vi "MGCC_StaEst_submain.vi"(0 "V_node":cdb[][](array[numeric]), 1 "I_node":cdb[][](array[numeric]), 2 "vbase":dbl=6928.4, 3 "sspn":dbl[][](array[numeric]), 4 "ssqn":dbl[][](array[numeric]), 5 "P_node":cdb[][](array[numeric]), 6 "ssvn":dbl[][](array[numeric]), 7 "Topology":dbl[][](array[numeric]), 9 "NumN":dbl, 11 "NumL":dbl, 12 "Ybus":cdb[][](array[numeric]), 15 "interrupt":dbl=1.0) -> (8 "VN":dbl[][](array[numeric]), 10 "error out":errorcluster, 14 "AN":dbl[][](array[numeric]))   [LabVIEW 2016]
doc: "-----------------------------------------------------------------------------------------------------------------------\nCopyright <2019> <The University of Tennessee at Knoxville and the University of Tennessee Research Foundation>\nThis software is released under BSD-3 \nhttps://opensource.org/licenses/BSD-3-Clause \nAdditional license options available at https://utrf.tennessee.edu/industry/sample-agreements/\n-----------------------------------------------------------------------------------------------------------------------"
uses:
  <vilib>/Utility/error.llb/Error Cluster From Error Code.vi
  Model Management/Global_MdlMgmt.vi
  <vilib>/imath/engines/lvmath2/RunTimeSupport/NIMS_Error if Not Equal.vi
  <instcachedir>/0/NIMS_Error if Not Equal_43252A79AD05436189442EC0C5E5AB8A.lvgen/NIMS_Error if Not Equal_43252A79AD05436189442EC0C5E5AB8A_000.vi
  <vilib>/imath/engines/lvmath2/RunTimeEngine/IndexRead/NIMS M(S,S).vi
  <instcachedir>/0/NIMS M(S,S)_AC51E74150A542F7991B9634C66F3096.lvgen/NIMS M(S,S)_AC51E74150A542F7991B9634C66F3096_001.vi
  <vilib>/imath/engines/lvmath2/RunTimeEngine/BuiltInFunctions/abs/NIMS_abs(signed).vi
  <instcachedir>/0/NIMS_abs(signed)_C4FCB8E6058B49B797C7C8D53CA5F6EC.lvgen/NIMS_abs(signed)_C4FCB8E6058B49B797C7C8D53CA5F6EC_002.vi
  <vilib>/imath/engines/lvmath2/RunTimeEngine/RunTimeType/NIMS_RunTimeType_From StrictType (excl LVString).vi
  <instcachedir>/0/NIMS_RunTimeType_From StrictType (excl LVString)_BBF44FB49F834B71AF7A14CCEDF8BECD.lvgen/NIMS_RunTimeType_From StrictType (excl LVString)_BBF44FB49F834B71AF7A14CCEDF8BECD_031.vi
  <vilib>/imath/engines/lvmath2/RunTimeEngine/Struct/NIMS_StructSetField.vi
  <vilib>/imath/engines/lvmath2/RunTimeEngine/ErrorHandling/NIMS_Create Error From Enums.vi
  <instcachedir>/0/NIMS_RunTimeType_From StrictType (excl LVString)_BBF44FB49F834B71AF7A14CCEDF8BECD.lvgen/NIMS_RunTimeType_From StrictType (excl LVString)_BBF44FB49F834B71AF7A14CCEDF8BECD_032.vi
  <vilib>/imath/engines/lvmath2/RunTimeEngine/Struct/NIMS_StructGetField.vi
  <vilib>/imath/engines/lvmath2/RunTimeEngine/RunTimeType/NIMS_RunTimeType_To Numeric.vi
  <instcachedir>/0/NIMS_RunTimeType_To Numeric_19D51BCABB82435A94073491761E42EE.lvgen/NIMS_RunTimeType_To Numeric_19D51BCABB82435A94073491761E42EE_010.vi
  <instcachedir>/0/NIMS_RunTimeType_To Numeric_19D51BCABB82435A94073491761E42EE.lvgen/NIMS_RunTimeType_To Numeric_19D51BCABB82435A94073491761E42EE_009.vi
  <instcachedir>/0/NIMS_RunTimeType_From StrictType (excl LVString)_BBF44FB49F834B71AF7A14CCEDF8BECD.lvgen/NIMS_RunTimeType_From StrictType (excl LVString)_BBF44FB49F834B71AF7A14CCEDF8BECD_000.vi
  <instcachedir>/0/NIMS_RunTimeType_To Numeric_19D51BCABB82435A94073491761E42EE.lvgen/NIMS_RunTimeType_To Numeric_19D51BCABB82435A94073491761E42EE_000.vi
  <vilib>/imath/engines/lvmath2/RunTimeEngine/IndexRead/NIMS M($,R2).vi
  <instcachedir>/0/NIMS M($,R2)_D9380E19261A4ADFB2D364AF6959C6EF.lvgen/NIMS M($,R2)_D9380E19261A4ADFB2D364AF6959C6EF_000.vi
  <vilib>/imathl/engines/lvmath/Functions/Error Handling/Create Error.vi
  <instcachedir>/0/NIMS_RunTimeType_From StrictType (excl LVString)_BBF44FB49F834B71AF7A14CCEDF8BECD.lvgen/NIMS_RunTimeType_From StrictType (excl LVString)_BBF44FB49F834B71AF7A14CCEDF8BECD_009.vi
  <vilib>/imath/engines/lvmath2/RunTimeEngine/BuiltInFunctions/imag/NIMS_imag(Complex).vi
  <instcachedir>/0/NIMS_imag(Complex)_3180D40D00C843A49C2B33397F857BF3.lvgen/NIMS_imag(Complex)_3180D40D00C843A49C2B33397F857BF3_001.vi
  <instcachedir>/0/NIMS_abs(signed)_C4FCB8E6058B49B797C7C8D53CA5F6EC.lvgen/NIMS_abs(signed)_C4FCB8E6058B49B797C7C8D53CA5F6EC_003.vi
  <vilib>/imath/engines/lvmath2/RunTimeEngine/BuiltInFunctions/angle/NIMS_angle.vi
  <instcachedir>/0/NIMS_angle_6DDAE2BD99E0421EB990B6436E94D88F.lvgen/NIMS_angle_6DDAE2BD99E0421EB990B6436E94D88F_001.vi
  <instcachedir>/0/NIMS_RunTimeType_To Numeric_19D51BCABB82435A94073491761E42EE.lvgen/NIMS_RunTimeType_To Numeric_19D51BCABB82435A94073491761E42EE_003.vi
  <instcachedir>/0/NIMS_abs(signed)_C4FCB8E6058B49B797C7C8D53CA5F6EC.lvgen/NIMS_abs(signed)_C4FCB8E6058B49B797C7C8D53CA5F6EC_005.vi
  <vilib>/imath/engines/lvmath2/RunTimeEngine/VariableToken/Support/NIMS_Matrix Boolean Index to I32 Index.vi
  <vilib>/imath/engines/lvmath2/RunTimeEngine/IndexReplace/NIMS M(V)=S.vi
  <instcachedir>/0/NIMS M(V)=S_F2304187E1344F60ABCBE5C5CC0920F9.lvgen/NIMS M(V)=S_F2304187E1344F60ABCBE5C5CC0920F9_000.vi
  <instcachedir>/0/NIMS M($,R2)_D9380E19261A4ADFB2D364AF6959C6EF.lvgen/NIMS M($,R2)_D9380E19261A4ADFB2D364AF6959C6EF_001.vi
  <instcachedir>/0/NIMS_RunTimeType_From StrictType (excl LVString)_BBF44FB49F834B71AF7A14CCEDF8BECD.lvgen/NIMS_RunTimeType_From StrictType (excl LVString)_BBF44FB49F834B71AF7A14CCEDF8BECD_024.vi
  LabVIEW Data/MathScriptVIs/MCStatic_36913153632_be44ae6048cc796b65fe61fbcc6124bb.vi
  <instcachedir>/0/MCStatic_36913153632_be44ae6048cc796b65fe61fbcc6124bb_299CCFB54962426892AA262595275464.lvgen/MCStatic_36913153632_be44ae6048cc796b65fe61fbcc6124bb_299CCFB54962426892AA262595275464_000.vi
  <instcachedir>/0/NIMS_RunTimeType_To Numeric_19D51BCABB82435A94073491761E42EE.lvgen/NIMS_RunTimeType_To Numeric_19D51BCABB82435A94073491761E42EE_008.vi
  <vilib>/imath/engines/lvmath2/RunTimeEngine/BuiltInFunctions/size/NIMS_I32=size(GRow,I32).vi
  <instcachedir>/0/NIMS_I32=size(GRow,I32)_ECB8D6BA8B644FAD9EC9BDD2BFE864D8.lvgen/NIMS_I32=size(GRow,I32)_ECB8D6BA8B644FAD9EC9BDD2BFE864D8_000.vi
  <vilib>/imath/engines/lvmath2/RunTimeEngine/RangeToken/NIMS_Range_R2 - Integer.vi
  <instcachedir>/0/NIMS_Range_R2 - Integer_89B873E74E6E489885E44F751DD9C6BF.lvgen/NIMS_Range_R2 - Integer_89B873E74E6E489885E44F751DD9C6BF_000.vi
  <vilib>/imath/engines/lvmath2/RunTimeEngine/CommandStatement/MC_CommandStatement_break.vi
  <vilib>/imath/engines/lvmath2/RunTimeEngine/IndexRead/NIMS M(S).vi
  <instcachedir>/0/NIMS M(S)_B826C018497E4940AE96BD27B540B6FB.lvgen/NIMS M(S)_B826C018497E4940AE96BD27B540B6FB_000.vi
  <vilib>/imath/engines/lvmath2/RunTimeEngine/MatrixToken/NIMS_MatrixToken_M_RV.vi
  <instcachedir>/0/NIMS_MatrixToken_M_RV_EE14907D4B194E829889005D2F556E9C.lvgen/NIMS_MatrixToken_M_RV_EE14907D4B194E829889005D2F556E9C_001.vi
  LabVIEW Data/MathScriptVIs/MCStatic_36913153632_768d10d24ec5cae2ef0a1ce42dd6f61b.vi
  <instcachedir>/0/MCStatic_36913153632_768d10d24ec5cae2ef0a1ce42dd6f61b_42FB18720A4D4D57895E758F2AD9E816.lvgen/MCStatic_36913153632_768d10d24ec5cae2ef0a1ce42dd6f61b_42FB18720A4D4D57895E758F2AD9E816_000.vi
  <vilib>/imath/engines/lvmath2/RunTimeEngine/RangeToken/NIMS_Range.vi
  <instcachedir>/0/NIMS_Range_A7C094595B484CA7AF10685B02D808ED.lvgen/NIMS_Range_A7C094595B484CA7AF10685B02D808ED_000.vi
  <instcachedir>/0/NIMS_RunTimeType_From StrictType (excl LVString)_BBF44FB49F834B71AF7A14CCEDF8BECD.lvgen/NIMS_RunTimeType_From StrictType (excl LVString)_BBF44FB49F834B71AF7A14CCEDF8BECD_010.vi
  <instcachedir>/0/NIMS_RunTimeType_To Numeric_19D51BCABB82435A94073491761E42EE.lvgen/NIMS_RunTimeType_To Numeric_19D51BCABB82435A94073491761E42EE_004.vi
  <vilib>/imath/engines/lvmath2/RunTimeEngine/BuiltInFunctions/length/NIMS_length(GV).vi
  <instcachedir>/0/NIMS_length(GV)_08A3D13377FD4E4B96F5795FBF3698FA.lvgen/NIMS_length(GV)_08A3D13377FD4E4B96F5795FBF3698FA_000.vi
  <vilib>/imath/engines/lvmath2/RunTimeEngine/BuiltInFunctions/size/NIMS_I32Row=size(GCol).vi
  <instcachedir>/0/NIMS_I32Row=size(GCol)_6F63159FA7824881BFA06400543D6D03.lvgen/NIMS_I32Row=size(GCol)_6F63159FA7824881BFA06400543D6D03_000.vi
  <vilib>/imath/engines/lvmath2/RunTimeEngine/RangeToken/NIMS_Range_R3 - Integer.vi
  <instcachedir>/0/NIMS_Range_R3 - Integer_A435E2FF893B4C718FD5055FE39FE2F6.lvgen/NIMS_Range_R3 - Integer_A435E2FF893B4C718FD5055FE39FE2F6_000.vi
  <vilib>/imath/engines/lvmath2/RunTimeEngine/IndexRead/NIMS V(S).vi
  <instcachedir>/0/NIMS V(S)_0488751826AF41519A22953C041130DC.lvgen/NIMS V(S)_0488751826AF41519A22953C041130DC_000.vi
  <vilib>/imath/engines/lvmath2/RunTimeEngine/IndexReplace/NIMS V(S)=S.vi
  <instcachedir>/0/NIMS V(S)=S_57E16554CB8B4B90AAB163894F717546.lvgen/NIMS V(S)=S_57E16554CB8B4B90AAB163894F717546_000.vi
  LabVIEW Data/MathScriptVIs/MCStatic_36913153632_1e6ad96140824169305d556de171d12e.vi
  <instcachedir>/0/MCStatic_36913153632_1e6ad96140824169305d556de171d12e_64F75552A8F844369C23CF330D52EDD5.lvgen/MCStatic_36913153632_1e6ad96140824169305d556de171d12e_64F75552A8F844369C23CF330D52EDD5_000.vi
  <instcachedir>/0/NIMS_Error if Not Equal_43252A79AD05436189442EC0C5E5AB8A.lvgen/NIMS_Error if Not Equal_43252A79AD05436189442EC0C5E5AB8A_001.vi
  <vilib>/imath/engines/lvmath2/RunTimeEngine/IndexRead/NIMS M(V,R2).vi
  <instcachedir>/0/NIMS M(V,R2)_C347351B41664C5DBDDF0EFBABEC5506.lvgen/NIMS M(V,R2)_C347351B41664C5DBDDF0EFBABEC5506_000.vi
  <vilib>/imath/engines/lvmath2/RunTimeEngine/ArithmeticOperatorToken/NIMS_ArithmeticOperator_times.vi
  <instcachedir>/0/NIMS_ArithmeticOperator_times_953B34F74CAC448FB707D816A29CC5F0.lvgen/NIMS_ArithmeticOperator_times_953B34F74CAC448FB707D816A29CC5F0_007.vi
  <vilib>/imath/engines/lvmath2/RunTimeEngine/BuiltInFunctions/reshapemx/NIMS_[GV]_reshapemx.vi
  <instcachedir>/0/NIMS_[GV]_reshapemx_314E456D64644EB191D4916921E89AA6.lvgen/NIMS_[GV]_reshapemx_314E456D64644EB191D4916921E89AA6_000.vi
  <vilib>/imath/engines/lvmath2/RunTimeEngine/IndexRead/NIMS M(V,S).vi
  <instcachedir>/0/NIMS M(V,S)_4A7282EC9BD94252BB5D44AC841A97D6.lvgen/NIMS M(V,S)_4A7282EC9BD94252BB5D44AC841A97D6_000.vi
  <vilib>/imath/engines/lvmath2/RunTimeEngine/IndexRead/NIMS M($,S).vi
  <instcachedir>/0/NIMS M($,S)_3E5749BBB62E49528D4765A77F1F6D98.lvgen/NIMS M($,S)_3E5749BBB62E49528D4765A77F1F6D98_000.vi
  <vilib>/imath/engines/lvmath2/RunTimeEngine/BuiltInFunctions/size/NIMS_I32Row=size(GRow).vi
  <instcachedir>/0/NIMS_I32Row=size(GRow)_E5C05C6B13124B29B774CC4F993D3C59.lvgen/NIMS_I32Row=size(GRow)_E5C05C6B13124B29B774CC4F993D3C59_000.vi
  <vilib>/imath/engines/lvmath2/RunTimeEngine/BuiltInFunctions/ones/NIMS_M=ones(I32V).vi
  <vilib>/imath/engines/lvmath2/RunTimeEngine/RowToken/NIMS_RowToken_M_M.vi
  <instcachedir>/0/NIMS_RowToken_M_M_968CDE3545E74ACDAEA4B48DE01EEECA.lvgen/NIMS_RowToken_M_M_968CDE3545E74ACDAEA4B48DE01EEECA_004.vi
  <vilib>/imath/engines/lvmath2/RunTimeEngine/BuiltInFunctions/diag/NIMS_diag.vi
  <instcachedir>/0/NIMS_diag_BAFF033CE85645D0951408836EA255EA.lvgen/NIMS_diag_BAFF033CE85645D0951408836EA255EA_003.vi
  <vilib>/imath/engines/lvmath2/RunTimeEngine/RowToken/NIMS_RowToken_CV_CV.vi
  <instcachedir>/0/NIMS_RowToken_CV_CV_5546A0B1CA2C4E49826F811B9C073FB0.lvgen/NIMS_RowToken_CV_CV_5546A0B1CA2C4E49826F811B9C073FB0_000.vi
  <vilib>/imath/engines/lvmath2/RunTimeEngine/BuiltInFunctions/zeros/NIMS_M=zeros(I32,I32).vi
  <vilib>/imath/engines/lvmath2/RunTimeEngine/RangeToken/NIMS_Range_R2 - Float.vi
  <instcachedir>/0/NIMS_Range_R2 - Float_590A1087448447AEB7F770FC082D3801.lvgen/NIMS_Range_R2 - Float_590A1087448447AEB7F770FC082D3801_000.vi
  <vilib>/imath/engines/lvmath2/RunTimeEngine/IndexReplace/NIMS M(S,S)=S.vi
  <instcachedir>/0/NIMS M(S,S)=S_98E40400474E4398B113AE20298B4F82.lvgen/NIMS M(S,S)=S_98E40400474E4398B113AE20298B4F82_000.vi
  LabVIEW Data/MathScriptVIs/MCStatic_36913153632_6298f8f6c83752723d2226ea016fc197.vi
  <instcachedir>/0/MCStatic_36913153632_6298f8f6c83752723d2226ea016fc197_3642FD24B40E4351BB90101570A96C12.lvgen/MCStatic_36913153632_6298f8f6c83752723d2226ea016fc197_3642FD24B40E4351BB90101570A96C12_000.vi
  LabVIEW Data/MathScriptVIs/MCStatic_36913153632_74b80caf5031e046e71450c869b25ac4.vi
  <instcachedir>/0/MCStatic_36913153632_74b80caf5031e046e71450c869b25ac4_EBBE0D165A1844C19D15217B3971A6C8.lvgen/MCStatic_36913153632_74b80caf5031e046e71450c869b25ac4_EBBE0D165A1844C19D15217B3971A6C8_000.vi
  <vilib>/imath/engines/lvmath2/RunTimeEngine/MatrixToken/NIMS_MatrixToken_M_M.vi
  <instcachedir>/0/NIMS_MatrixToken_M_M_DF273B0CC20F424BBF1EDA9F4E71C841.lvgen/NIMS_MatrixToken_M_M_DF273B0CC20F424BBF1EDA9F4E71C841_004.vi
  <vilib>/imath/engines/lvmath2/RunTimeEngine/IndexReplace/NIMS M($,V)=S.vi
  <instcachedir>/0/NIMS M($,V)=S_8FF4B0FF94A24B3598424F2A899DBD06.lvgen/NIMS M($,V)=S_8FF4B0FF94A24B3598424F2A899DBD06_000.vi
  LabVIEW Data/MathScriptVIs/MCStatic_36913153632_b1439afdde66222fcd04c55d7a6778ce.vi
  <instcachedir>/0/MCStatic_36913153632_b1439afdde66222fcd04c55d7a6778ce_EEE05774F8294989AC0FB7279B922BFB.lvgen/MCStatic_36913153632_b1439afdde66222fcd04c55d7a6778ce_EEE05774F8294989AC0FB7279B922BFB_000.vi
  LabVIEW Data/MathScriptVIs/MCStatic_36913153632_4de716850640586bd02f98b625ef993e.vi
  <instcachedir>/0/MCStatic_36913153632_4de716850640586bd02f98b625ef993e_4E7D4A7640E146149C2F9063A07B5FB8.lvgen/MCStatic_36913153632_4de716850640586bd02f98b625ef993e_4E7D4A7640E146149C2F9063A07B5FB8_000.vi
  <vilib>/imath/engines/lvmath2/RunTimeEngine/ArithmeticOperatorToken/NIMS_ArithmeticOperator_minus.vi
  <instcachedir>/0/NIMS_ArithmeticOperator_minus_E3B65B1D26A44BB184AFDC5B3F458E3D.lvgen/NIMS_ArithmeticOperator_minus_E3B65B1D26A44BB184AFDC5B3F458E3D_003.vi
  <vilib>/imath/engines/lvmath2/RunTimeEngine/ArithmeticOperatorToken/NIMS_ArithmeticOperator_rightdivmx.vi
  <instcachedir>/0/NIMS_ArithmeticOperator_rightdivmx_0DBBD6F2821B4AB59571CD9AB2DE9D62.lvgen/NIMS_ArithmeticOperator_rightdivmx_0DBBD6F2821B4AB59571CD9AB2DE9D62_000.vi
  <vilib>/imath/engines/lvmath2/RunTimeEngine/ArithmeticOperatorToken/NIMS_ArithmeticOperator_multmx(M,CV).vi
  <instcachedir>/0/NIMS_ArithmeticOperator_multmx(M,CV)_EE734FC8520844C9A7CC1A67008668A3.lvgen/NIMS_ArithmeticOperator_multmx(M,CV)_EE734FC8520844C9A7CC1A67008668A3_000.vi
  <vilib>/imath/engines/lvmath2/RunTimeEngine/ArithmeticOperatorToken/NIMS_ArithmeticOperator_multmx.vi
  <instcachedir>/0/NIMS_ArithmeticOperator_multmx_4A56FE5C615140CE835D4DB5891BF065.lvgen/NIMS_ArithmeticOperator_multmx_4A56FE5C615140CE835D4DB5891BF065_004.vi
  <vilib>/imath/engines/lvmath2/RunTimeEngine/BuiltInFunctions/pinv/NIMS_pinv.vi
  <instcachedir>/0/NIMS_pinv_206F0700CF75499C820074BA4F1FFC36.lvgen/NIMS_pinv_206F0700CF75499C820074BA4F1FFC36_000.vi
  <vilib>/imath/engines/lvmath2/RunTimeEngine/ErrorHandling/NIMS_Error From Error Code.vi
  LabVIEW Data/MathScriptVIs/MCStatic_36913153632_4a49c84bbcd428c212b20195cbe8b035.vi
  <instcachedir>/0/MCStatic_36913153632_4a49c84bbcd428c212b20195cbe8b035_991BF795119A46088146E750DEF0BE67.lvgen/MCStatic_36913153632_4a49c84bbcd428c212b20195cbe8b035_991BF795119A46088146E750DEF0BE67_000.vi
  LabVIEW Data/MathScriptVIs/MCStatic_36913153632_a7ddd08330f9b3077b19931b3d4ed570.vi
  <instcachedir>/0/MCStatic_36913153632_a7ddd08330f9b3077b19931b3d4ed570_A5488D48717747F080A6F4A94BE5B924.lvgen/MCStatic_36913153632_a7ddd08330f9b3077b19931b3d4ed570_A5488D48717747F080A6F4A94BE5B924_000.vi
  <instcachedir>/0/NIMS_ArithmeticOperator_minus_E3B65B1D26A44BB184AFDC5B3F458E3D.lvgen/NIMS_ArithmeticOperator_minus_E3B65B1D26A44BB184AFDC5B3F458E3D_002.vi
  <vilib>/imath/engines/lvmath2/RunTimeEngine/BuiltInFunctions/max/1 input/NIMS_max(RM).vi
  <instcachedir>/0/NIMS_max(RM)_358AE92FF7FA4D91BF0D9DEC69043403.lvgen/NIMS_max(RM)_358AE92FF7FA4D91BF0D9DEC69043403_000.vi
  <vilib>/imath/engines/lvmath2/RunTimeEngine/ArithmeticOperatorToken/NIMS_ArithmeticOperator_plus.vi
  <instcachedir>/0/NIMS_ArithmeticOperator_plus_0120E0498A0F4B4B9BDCAC2554767A4E.lvgen/NIMS_ArithmeticOperator_plus_0120E0498A0F4B4B9BDCAC2554767A4E_003.vi
  <vilib>/imath/engines/lvmath2/RunTimeEngine/VariableToken/NIMS_VariableToken_CondDefined.vi
  <instcachedir>/0/NIMS_VariableToken_CondDefined_06E9DA95BD4D46A6BA55EC651A891960.lvgen/NIMS_VariableToken_CondDefined_06E9DA95BD4D46A6BA55EC651A891960_001.vi
  <vilib>/imath/engines/lvmath2/RunTimeEngine/IndexRead/NIMS M(V).vi
  <instcachedir>/0/NIMS M(V)_948FAC22C1C943948B75DA6190348614.lvgen/NIMS M(V)_948FAC22C1C943948B75DA6190348614_005.vi
  <vilib>/imath/engines/lvmath2/RunTimeEngine/BuiltInFunctions/reshapemx/NIMS_[GM]_reshapemx.vi
  <instcachedir>/0/NIMS_[GM]_reshapemx_500BD31B48F5434EA23B2056DCB44201.lvgen/NIMS_[GM]_reshapemx_500BD31B48F5434EA23B2056DCB44201_000.vi
  <instcachedir>/0/NIMS_ArithmeticOperator_plus_0120E0498A0F4B4B9BDCAC2554767A4E.lvgen/NIMS_ArithmeticOperator_plus_0120E0498A0F4B4B9BDCAC2554767A4E_010.vi
  <instcachedir>/0/NIMS_VariableToken_CondDefined_06E9DA95BD4D46A6BA55EC651A891960.lvgen/NIMS_VariableToken_CondDefined_06E9DA95BD4D46A6BA55EC651A891960_004.vi
  <instcachedir>/0/NIMS_VariableToken_CondDefined_06E9DA95BD4D46A6BA55EC651A891960.lvgen/NIMS_VariableToken_CondDefined_06E9DA95BD4D46A6BA55EC651A891960_005.vi
  <vilib>/imath/engines/lvmath/Functions/Error Handling/MergeErrorsWrapper.vi
  <vilib>/imath/engines/lvmath2/RunTimeEngine/NodeEndStatement/NIMS_NodeEndStatement_Output.vi
  <instcachedir>/0/NIMS_NodeEndStatement_Output_53EC0D466D134D7ABD903AC30B43404B.lvgen/NIMS_NodeEndStatement_Output_53EC0D466D134D7ABD903AC30B43404B_002.vi
  <instcachedir>/0/NIMS_NodeEndStatement_Output_53EC0D466D134D7ABD903AC30B43404B.lvgen/NIMS_NodeEndStatement_Output_53EC0D466D134D7ABD903AC30B43404B_005.vi
  <instcachedir>/0/NIMS_NodeEndStatement_Output_53EC0D466D134D7ABD903AC30B43404B.lvgen/NIMS_NodeEndStatement_Output_53EC0D466D134D7ABD903AC30B43404B_025.vi
  <instcachedir>/0/NIMS_NodeEndStatement_Output_53EC0D466D134D7ABD903AC30B43404B.lvgen/NIMS_NodeEndStatement_Output_53EC0D466D134D7ABD903AC30B43404B_011.vi
  <instcachedir>/0/NIMS_NodeEndStatement_Output_53EC0D466D134D7ABD903AC30B43404B.lvgen/NIMS_NodeEndStatement_Output_53EC0D466D134D7ABD903AC30B43404B_024.vi
  <instcachedir>/0/NIMS_NodeEndStatement_Output_53EC0D466D134D7ABD903AC30B43404B.lvgen/NIMS_NodeEndStatement_Output_53EC0D466D134D7ABD903AC30B43404B_003.vi
  <instcachedir>/0/NIMS_NodeEndStatement_Output_53EC0D466D134D7ABD903AC30B43404B.lvgen/NIMS_NodeEndStatement_Output_53EC0D466D134D7ABD903AC30B43404B_001.vi
  <instcachedir>/0/NIMS_NodeEndStatement_Output_53EC0D466D134D7ABD903AC30B43404B.lvgen/NIMS_NodeEndStatement_Output_53EC0D466D134D7ABD903AC30B43404B_023.vi
  <instcachedir>/0/NIMS_NodeEndStatement_Output_53EC0D466D134D7ABD903AC30B43404B.lvgen/NIMS_NodeEndStatement_Output_53EC0D466D134D7ABD903AC30B43404B_022.vi
  <instcachedir>/0/NIMS_NodeEndStatement_Output_53EC0D466D134D7ABD903AC30B43404B.lvgen/NIMS_NodeEndStatement_Output_53EC0D466D134D7ABD903AC30B43404B_021.vi
  <instcachedir>/0/NIMS_NodeEndStatement_Output_53EC0D466D134D7ABD903AC30B43404B.lvgen/NIMS_NodeEndStatement_Output_53EC0D466D134D7ABD903AC30B43404B_020.vi
  <instcachedir>/0/NIMS_NodeEndStatement_Output_53EC0D466D134D7ABD903AC30B43404B.lvgen/NIMS_NodeEndStatement_Output_53EC0D466D134D7ABD903AC30B43404B_019.vi
  <instcachedir>/0/NIMS_NodeEndStatement_Output_53EC0D466D134D7ABD903AC30B43404B.lvgen/NIMS_NodeEndStatement_Output_53EC0D466D134D7ABD903AC30B43404B_018.vi
  <instcachedir>/0/NIMS_NodeEndStatement_Output_53EC0D466D134D7ABD903AC30B43404B.lvgen/NIMS_NodeEndStatement_Output_53EC0D466D134D7ABD903AC30B43404B_017.vi
  <instcachedir>/0/NIMS_NodeEndStatement_Output_53EC0D466D134D7ABD903AC30B43404B.lvgen/NIMS_NodeEndStatement_Output_53EC0D466D134D7ABD903AC30B43404B_004.vi
  <instcachedir>/0/NIMS_NodeEndStatement_Output_53EC0D466D134D7ABD903AC30B43404B.lvgen/NIMS_NodeEndStatement_Output_53EC0D466D134D7ABD903AC30B43404B_027.vi
  <vilib>/imath/engines/lvmath2/RunTimeEngine/ErrorHandling/NIMS_Finalize Error.vi
  <vilib>/imath/engines/lvmath2/RunTimeEngine/RelationalOperatorToken/NIMS_Relational_Operator_Eq.vi
  <instcachedir>/0/NIMS_Relational_Operator_Eq_FD198F059617437A8A02361002FCA645.lvgen/NIMS_Relational_Operator_Eq_FD198F059617437A8A02361002FCA645_003.vi
  <instcachedir>/0/NIMS_NodeEndStatement_Output_53EC0D466D134D7ABD903AC30B43404B.lvgen/NIMS_NodeEndStatement_Output_53EC0D466D134D7ABD903AC30B43404B_015.vi
  <vilib>/ErrorRing/Error Ring.xnode
  cequ.m
  cjoc.m
  idx2pha.m
  pha2idx.m
  pnequ.m
  pnjoc.m
  vnequ.m
  vnjoc.m
  zeroinjec.m
  <instcachedir>/0/MCStatic_36913153632_4de716850640586bd02f98b625ef993e_4E7D4A7640E146149C2F9063A07B5FB8.lvgen/MCStatic_36913153632_4de716850640586bd02f98b625ef993e_4E7D4A7640E146149C2F9063A07B5FB8_001.vi
  <instcachedir>/0/MCStatic_36913153632_6298f8f6c83752723d2226ea016fc197_3642FD24B40E4351BB90101570A96C12.lvgen/MCStatic_36913153632_6298f8f6c83752723d2226ea016fc197_3642FD24B40E4351BB90101570A96C12_001.vi
  <instcachedir>/0/MCStatic_36913153632_74b80caf5031e046e71450c869b25ac4_EBBE0D165A1844C19D15217B3971A6C8.lvgen/MCStatic_36913153632_74b80caf5031e046e71450c869b25ac4_EBBE0D165A1844C19D15217B3971A6C8_001.vi
  <instcachedir>/0/MCStatic_36913153632_a7ddd08330f9b3077b19931b3d4ed570_A5488D48717747F080A6F4A94BE5B924.lvgen/MCStatic_36913153632_a7ddd08330f9b3077b19931b3d4ed570_A5488D48717747F080A6F4A94BE5B924_001.vi
  <instcachedir>/0/MCStatic_36913153632_b1439afdde66222fcd04c55d7a6778ce_EEE05774F8294989AC0FB7279B922BFB.lvgen/MCStatic_36913153632_b1439afdde66222fcd04c55d7a6778ce_EEE05774F8294989AC0FB7279B922BFB_001.vi
panel:
  out "H":dbl[][](array[numeric])
  out "InitialValue":dbl[](array[numeric])
  out "StateVar":dbl[][](array[numeric])
  out "Weight":dbl[][](array[numeric])
  out "Num":T1
  out "B":dbl[][](array[numeric])
  out "MeaPha":T2
  out "Loc":cluster{"Zeroinj":i32[][], "Line":dbl[][]}
  out "pha_rupter":i32[][](array[numeric])
  out "puTrue":T3
  out "Mea":T2
  out "measure":dbl[](array[numeric])
  out "G":dbl[][](array[numeric])
  out "V_node 2":cdb[][](array[numeric])
  out "MeaIdx":cluster{"PN":dbl[], "QN":dbl[], "VN":dbl[]}
  out "idx_rupter":dbl[](array[numeric])
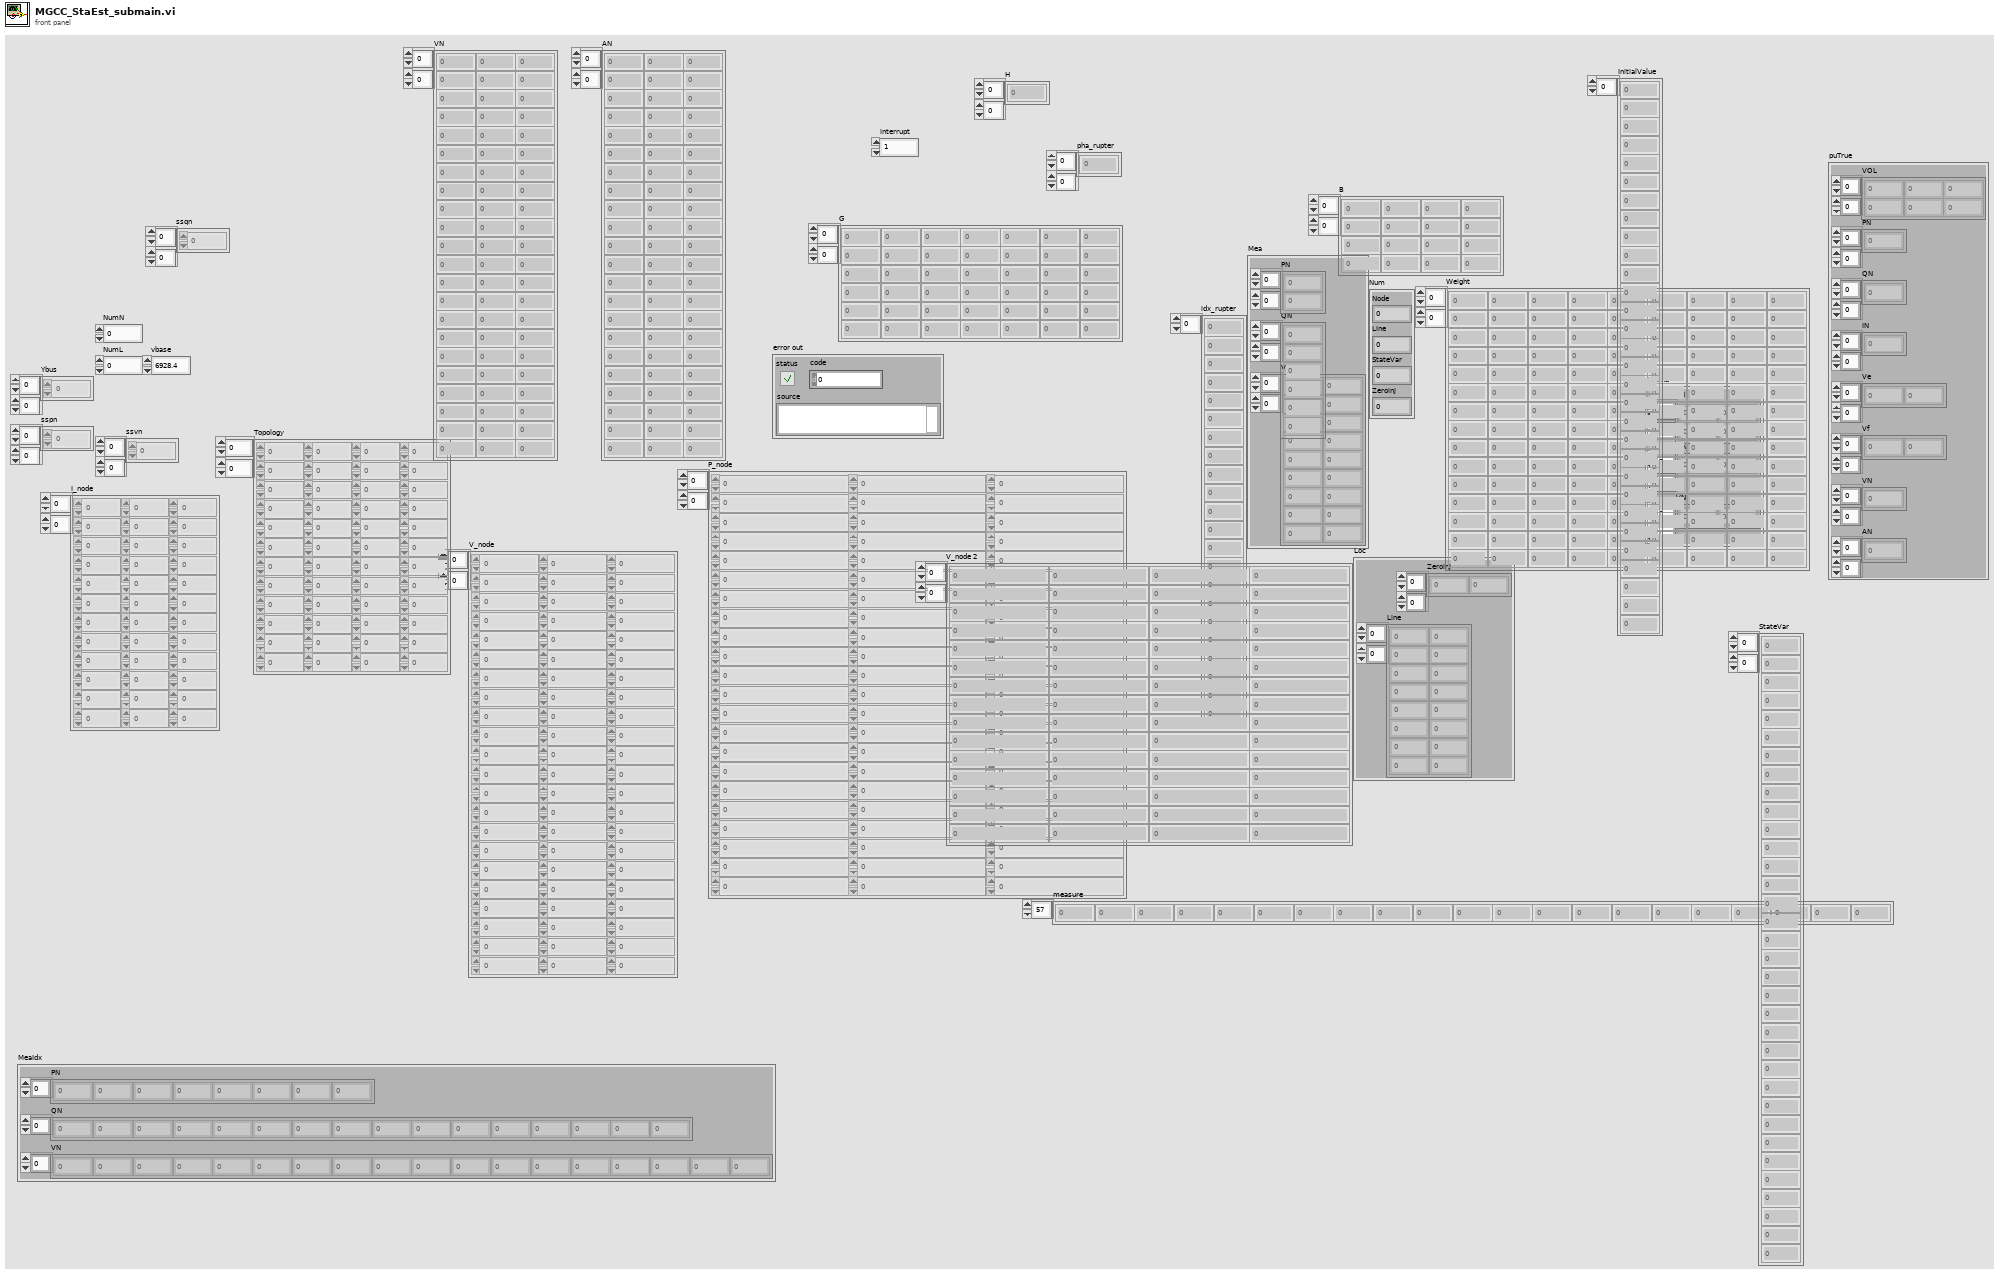
[diagram p1: front panel]
types:
  T1 = cluster{"Node":dbl, "Line":dbl, "StateVar":i32, "Zeroinj":i32}
  T2 = cluster{"PN":dbl[][], "QN":dbl[][], "VN":dbl[][]}
  T3 = cluster{"VOL":cdb[][], "PN":dbl[][], "QN":dbl[][], "IN":dbl[][], "Ve":dbl[][], "Vf":dbl[][], "VN":dbl[][], "AN":dbl[][]}
  T4 = cluster{"Ve":dbl[][], "Vf":dbl[][], "VOL":cdb[][], "AN":dbl[][], "VN":dbl[][]}
  T5 = cluster{"Sbase":dbl, "Vbase":i32, "Ibase":dbl, "Ybase":dbl}
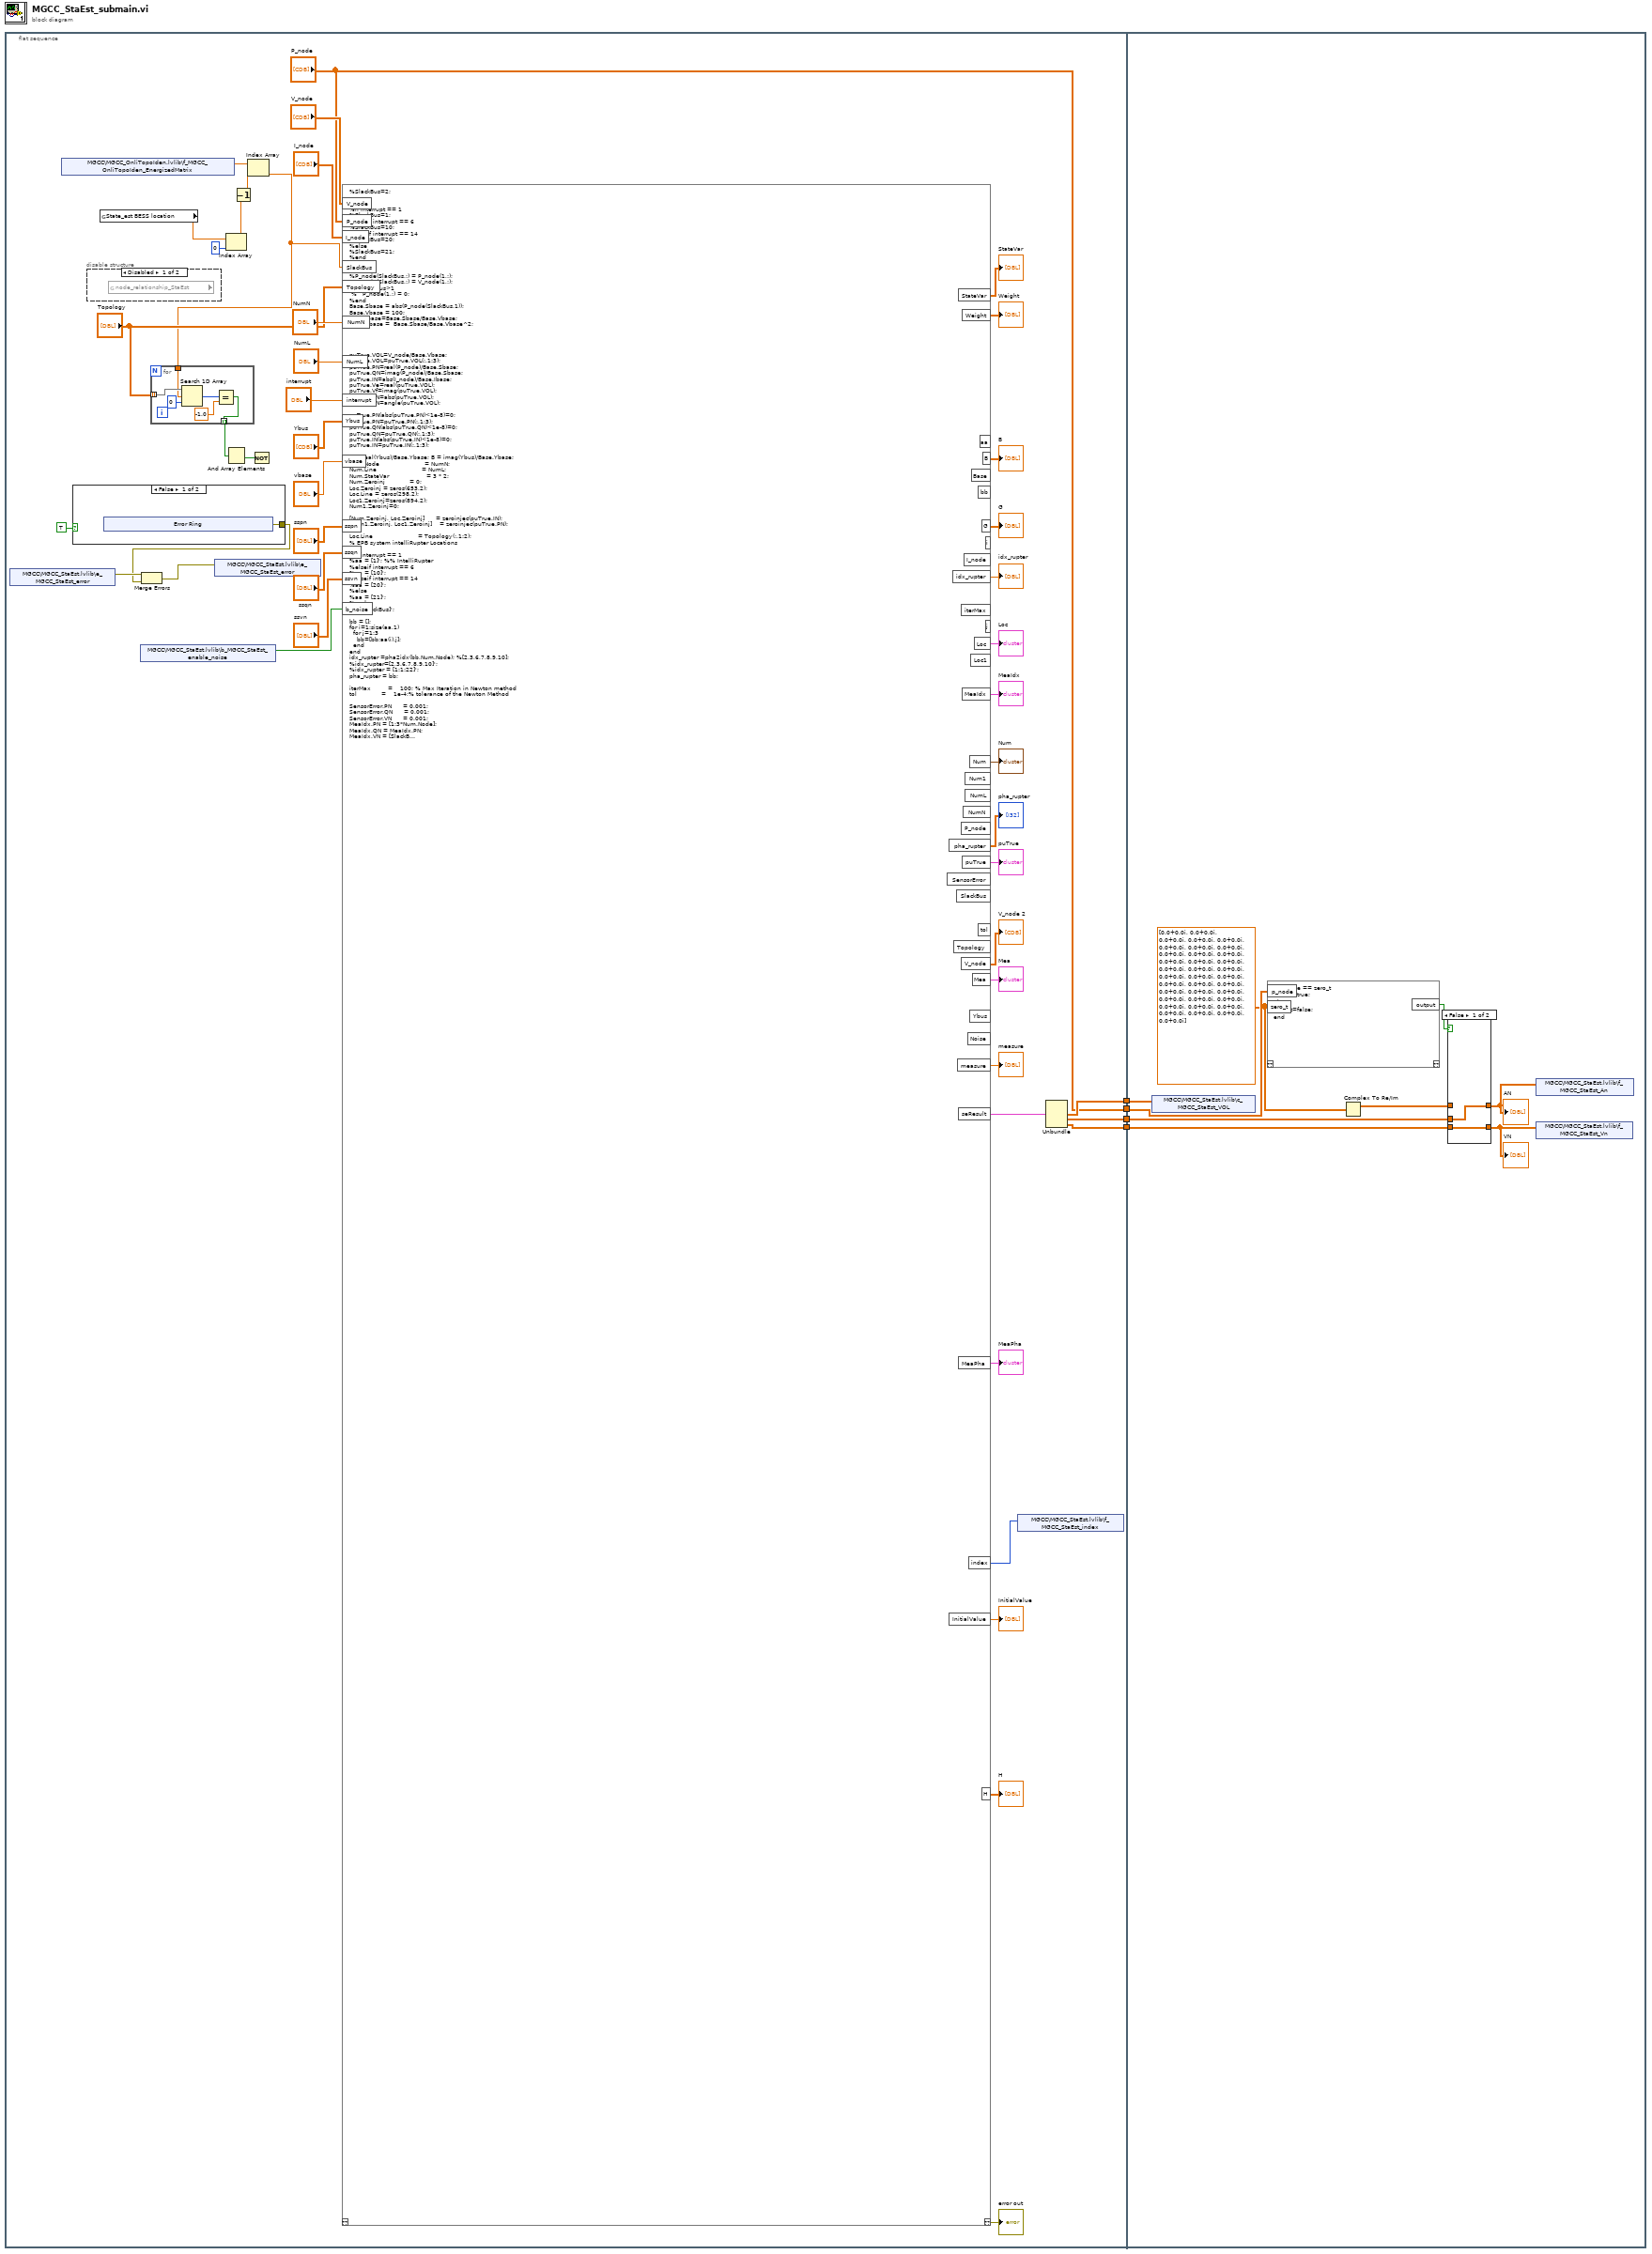
[diagram p0: block diagram]
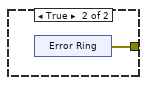
[diagram p2: hidden frame]
diagram:
  n1 = flat-sequence {
    tunnel: [w37] -> w4
    tunnel: ["P_node"] -> w3
    tunnel: [w22] -> w2
    tunnel: [w21] -> w1
    tunnel: w4 -> [w3950]
    tunnel: w3 -> [w3949]
    tunnel: w2 -> [w3946]
    tunnel: w1 -> [w3948]
    frame #0 {
      n2 = shared-variable "MGCC\\MGCC_StaEst.lvlib\\e_MGCC_StaEst_error"() -> (w8:errorcluster)  [unwired: 1 in, 1 out]
      n3 = shared-variable "MGCC\\MGCC_OnliTopoIden.lvlib\\f_MGCC_OnliTopoIden_EnergizedMatrix"() -> (w18:dbl[])  [unwired: 1 in, 1 out]
      n4 = case shown="False" TRUE {
        tunnel: [w52 w58] -> w6
        frame False {
          n5 = xnode "Error Ring"() -> ("error out"=w52:errorcluster)
        }
        frame True {
          n6 = xnode "Error Ring"() -> ("error out"=w58:errorcluster)
        }
      }
      n7 = disable-structure shown="Disabled" {
        frame Disabled {
          n8 = global read "Global_MdlMgmt.vi" "node_relationship_StaEst"() -> ()  [unwired: 1 out]
        }
        frame Enabled {
        }
      }
      n9 = global read "Global_MdlMgmt.vi" "State_est BESS location"() -> (w17:dbl[])
      n10 = shared-variable "MGCC\\MGCC_StaEst.lvlib\\b_MGCC_StaEst_enable_noise"() -> (w38:bool)  [unwired: 1 in, 1 out]
      n11 = Merge Errors(w8, w6) -> (w7:errorcluster)
      n12 = shared-variable "MGCC\\MGCC_StaEst.lvlib\\e_MGCC_StaEst_error"(w7) -> ()  [unwired: 1 in, 1 out]
      n13 = Index Array(array=w17, index=0) -> (element=w15:dbl)
      n14 = Decrement(x=w15) -> (x-1=w14:dbl)
      n15 = Index Array(array=w18, index=w14) -> (element=w11:dbl)
      n16 = for {
        tunnel: "Topology" -> [w65] mode=indexing
        tunnel: w11 -> [w64]
        tunnel: [w60] -> w10 mode=indexing
        n17 = Search 1D Array(1D array=w65, element=w64, start index (0)=0) -> (index of element=w61:i32)
        n18 = Equal?(x=w61, y=-1.0) -> (x = y?=w60:bool)
      }
      n19 = And Array Elements(Boolean array=w10) -> (logical AND=w9:bool)
      n20 = Not(x=w9) -> ()  [unwired: 1 out]
      n21 = mathscript code="%SlackBus=2;\n\n\n%if interrupt == 1\n%SlackBus=1;\n%elseif interrupt == 6\n%SlackBus=10;\n%elseif interrupt == 14\n%SlackBus=20;\n%else\n%SlackBus=21;\n%end\n\n\n%P_node(SlackBus,:) = P_node(1,:);\n%V_node(SlackBus,:) = V_node(1,:);\n%if SlackBus>1\n %   P_node(1,:) = 0;\n%end\nBase.Sbase = abs(P_node(SlackBus,1));\nBase.Vbase = 100;\nBase.Ibase=Base.Sbase/Base.Vbase;\nBase.Ybase =  Base.Sbase/Base.Vbase^2;\n\n\n\n\npuTrue.VOL=V_node/Base.Vbase;\npuTrue.VOL=puTrue.VOL(:,1:3);\npuTrue.PN=real(P_node)/Base.Sbase;\npuTrue.QN=imag(P_node)/Base.Sbase;\npuTrue.IN=abs(I_node)/Base.Ibase;\npuTrue.Ve=real(puTrue.VOL);\npuTrue.Vf=imag(puTrue.VOL); \npuTrue.VN=abs(puTrue.VOL);\npuTrue.AN=angle(puTrue.VOL);\n\npuTrue.PN(abs(puTrue.PN)<1e-8)=0;\npuTrue.PN=puTrue.PN(:,1:3);\npuTrue.QN(abs(puTrue.QN)<1e-8)=0;\npuTrue.QN=puTrue.QN(:,1:3);\npuTrue.IN(abs(puTrue.IN)<1e-8)=0;\npuTrue.IN=puTrue.IN(:,1:3);\n\nG = real(Ybus)/Base.Ybase; B = imag(Ybus)/Base.Ybase;\nNum.Node                        = NumN;\nNum.Line                        = NumL;\nNum.StateVar                    = 3 * 2;  \nNum.Zeroinj             = 0;\nLoc.Zeroinj = zeros(653,2);\nLoc.Line = zeros(298,2);\nLoc1.Zeroinj=zeros(894,2);\nNum1.Zeroinj=0;\n\n[Num.Zeroinj, Loc.Zeroinj]      = zeroinjec(puTrue.IN);\n[Num1.Zeroinj, Loc1.Zeroinj]    = zeroinjec(puTrue.PN);\n\nLoc.Line                        = Topology(:,1:2);\n% EPB system intelliRupter Locations\n\n%if interrupt == 1\n%aa = [1]'; %% IntelliRupter\n%elseif interrupt == 6\n%aa = [10]';\n%elseif interrupt == 14\n%aa = [20]';\n%else\n%aa = [21]';\n%end\naa=[SlackBus]';\n\nbb = [];\nfor i=1:size(aa,1)\n  for j=1:3\n    bb=[bb;aa(i),j];\n  end\nend\nidx_rupter =pha2idx(bb,Num.Node); %[2,3,6,7,8,9,10];\n%idx_rupter=[2,3,6,7,8,9,10]';\n%idx_rupter = [1:1:22]';\npha_rupter = bb;\n\niterMax         =    100; % Max Iteration in Newton method\ntol             =    1e-4;% tolerance of the Newton Method\n\nSensorError.PN      = 0.001;\nSensorError.QN      = 0.001;\nSensorError.VN      = 0.001;\nMeaIdx.PN = [1:3*Num.Node];\nMeaIdx.QN = MeaIdx.PN;\nMeaIdx.VN = [SlackBus:Num.Node:3*Num.Node];\n%MeaIdx.VN = [1,13,25];\n%MeaIdx.VN = [MeaIdx.VN,idx_rupter];\n\ntemp_size=length(MeaIdx.VN);\nfor i=1:1:size(idx_rupter)\n     MeaIdx.VN(i+temp_size) = idx_rupter(i); \nend\n\nMeaPha.PN = idx2pha(MeaIdx.PN,Num.Node);\nMeaPha.QN = idx2pha(MeaIdx.QN,Num.Node);\nMeaPha.VN = idx2pha(MeaIdx.VN,Num.Node);\n%% Step 4: Creat measure with noise\n%Noise.PN = zeros(10,3)+1+rand(10,3)*0.1;\n%Noise.QN = zeros(10,3)+1+rand(10,3)*0.1;\n%Noise.VN = zeros(10,3)+1+rand(10,3)*0.1;\n\nNoise.PN = sspn';\nNoise.QN = ssqn';\nNoise.VN = ssvn';\nNoise.PN = Noise.PN(1:Num.Node ,1:3);\nNoise.QN = Noise.QN(1:Num.Node ,1:3);\nNoise.VN = Noise.VN(1:Num.Node ,1:3);\nif b_noise\nMea.PN  = puTrue.PN.* Noise.PN; \nMea.QN  = puTrue.QN.* Noise.QN;\nMea.VN  = puTrue.VN.^2.* Noise.VN;\nelse\nMea.PN  = puTrue.PN;% .* Noise.PN; \nMea.QN  = puTrue.QN;% .* Noise.QN;\nMea.VN  = puTrue.VN.^2 ;%.* Noise.VN;\nend\nMea.PN  = reshape(Mea.PN,3*Num.Node,1);\nMea.QN  = reshape(Mea.QN,3*Num.Node,1);\nMea.VN  = reshape(Mea.VN,3*Num.Node,1);\n\n\nmeasure = [Mea.PN(MeaIdx.PN,1); Mea.QN(MeaIdx.QN,1);Mea.VN(MeaIdx.VN,1)];\nmeasure = measure(:,1);\n\nWPN = SensorError.PN*ones(size(MeaIdx.PN));\nWQN = SensorError.QN*ones(size(MeaIdx.QN));\nWVN = SensorError.VN*ones(size(MeaIdx.VN));\n\nWeight =diag([WPN.^2,WQN.^2,WVN.^2]);\n\nVe1 = reshape(puTrue.Ve,3*Num.Node,1);\nVf1 = reshape(puTrue.Vf,3*Num.Node,1);\nVV1 = [Ve1,Vf1];\nStateVar_true= reshape(VV1',Num.StateVar * Num.Node,1);\n       \nVe_temp = zeros(Num.Node,3);\nVf_temp = zeros(Num.Node,3);\n\nfor i=1:Num.Node\n    for d=1:3\n %       if puTrue.Ve(i,d) == 0\n %           Ve_temp(i,d)=0;Vf_temp(i,d)=0;\n %       else\n            if d==1\n                Ve_temp(i,d)=cos(0*pi/180); %1.0167*\n                Vf_temp(i,d)=-sin(0*pi/180);\n            end\n            if d==2\n                Ve_temp(i,d)=cos(-120*pi/180);\n                Vf_temp(i,d)=-sin(-120*pi/180);\n            end\n            if d==3\n                Ve_temp(i,d)=cos(120*pi/180);\n                Vf_temp(i,d)=-sin(120*pi/180);            \n            end\n        end\n    end\n%end\n\nVe1p = reshape(Ve_temp,3*Num.Node,1);\nVf1p = reshape(Vf_temp,3*Num.Node,1);\nVV1p = [Ve1p,-Vf1p];\nInitialValue= reshape(VV1p',Num.StateVar*Num.Node,1);\nStateVar = reshape(VV1p',Num.StateVar*Num.Node,1);\n\n\nfor i = 1:iterMax\n  % Jocobian matrix\n  [joc_pn,joc_qn] = pnjoc(Num,StateVar,MeaPha,B,G);\n  joc_vn          = vnjoc(Num,StateVar,MeaPha);\n  H = [joc_pn;joc_qn;joc_vn];\n  H(:,2*SlackBus:2*Num.Node:end)=0;   \n  H(:,2*SlackBus-1:2*Num.Node:end)=0; \nindex=i;\n  % MeaEqu\n  [equ_pn,equ_qn] = pnequ(Num,StateVar,MeaPha,B,G);\n  equ_vn = vnequ(Num,StateVar,MeaPha);\n  MeaEqu = [equ_pn;equ_qn;equ_vn];\n  \n  delta_z = measure-MeaEqu;\n  G2 = H'/Weight*delta_z;\n  G3 = H'/Weight*H;    \n  Ginv = pinv(G3);\n  \n  [joc_c,joc_d] = cjoc(Num,B,G,Loc);\n  C = [joc_c;joc_d];\n  C(:,2*SlackBus:2*Num.Node:end)=0;\n  C(:,2*SlackBus-1:2*Num.Node:end)=0;\n  [equ_c,equ_d] = cequ(Num,StateVar,B,G,Loc);\n  delta_c = [-equ_c;-equ_d];  \n  C_temp1 = C*Ginv*C';\n  C_temp2 = pinv(C_temp1);\n  deltaX = Ginv * G2 -Ginv*C'*(C_temp2*(C*Ginv*G2-delta_c)); \n\n  deltaX(abs(deltaX)<1e-8)=0;\n  tol_temp = max(abs(deltaX));\nindex=i;\n  if tol_temp < tol\n      break;\n  end\n  StateVar = StateVar + deltaX;\nend\n\ntempVe=StateVar(1:2:6*Num.Node-1);\ntempVf=StateVar(2:2:6*Num.Node);\nseResult.Ve=reshape(tempVe,Num.Node,3);\nseResult.Vf=reshape(tempVf,Num.Node,3);\nseResult.VOL=seResult.Ve+1i*seResult.Vf;\nseResult.AN=angle(seResult.VOL);\nseResult.VN=abs(seResult.VOL);\n\n%VN = abs(seResult.VN - 1); \n%AN = seResult.AN; \n%VOL = cos(AN).*VN + i*sin(AN).*VN;"("V_node"="V_node", "P_node"="P_node", "I_node"="I_node", "NumN"="NumN", "NumL"="NumL", "Ybus"="Ybus", "sspn"="sspn", "ssqn"="ssqn", "ssvn"="ssvn", "SlackBus"=w11, "Topology"="Topology", "vbase"="vbase", "b_noise"=w38, "interrupt"="interrupt") -> ("??"=→"error out":errorcluster, "B"=→"B":dbl[][], "G"=→"G":dbl[][], "idx_rupter"=→"idx_rupter":dbl[], "Loc"=→"Loc":cluster{"Zeroinj":i32[][], "Line":dbl[][]}, "MeaIdx"=→"MeaIdx":cluster{"PN":dbl[], "QN":dbl[], "VN":dbl[]}, "Num"=→"Num":T1, "pha_rupter"=→"pha_rupter":dbl[][], "puTrue"=→"puTrue":T3, "V_node"=→"V_node 2":cdb[][], "Mea"=→"Mea":T2, "measure"=→"measure":dbl[], "seResult"=w51:T4, "index"=w19:i32, "MeaPha"=→"MeaPha":T2, "Weight"=→"Weight":dbl[][], "StateVar"=→"StateVar":dbl[][], "InitialValue"=→"InitialValue":dbl[], "H"=→"H":dbl[][])  [unwired: 1 in, 18 out]
      n22 = shared-variable "MGCC\\MGCC_StaEst.lvlib\\f_MGCC_StaEst_index"(w19) -> ()  [unwired: 1 in, 1 out]
      n23 = Unbundle(w51) -> ("VOL"=w37:cdb[][], "AN"=w22:dbl[][], "VN"=w21:dbl[][])  [unwired: 2 out]
    }
    frame #1 {
      w3944 = cdb[][] [[0.0+0.0i, 0.0+0.0i, 0.0+0.0i], [0.0+0.0i, 0.0+0.0i, 0.0+0.0i], [0.0+0.0i, 0.0+0.0i, 0.0+0.0i], [0.0+0.0i, 0.0+0.0i, 0.0+0.0i], [0.0+0.0i, 0.0+0.0i, 0.0+0.0i], [0.0+0.0i, 0.0+0.0i, 0.0+0.0i], [0.0+0.0i, 0.0+0.0i, 0.0+0.0i], [0.0+0.0i, 0.0+0.0i, 0.0+0.0i], [0.0+0.0i, 0.0+0.0i, 0.0+0.0i], [0.0+0.0i, 0.0+0.0i, 0.0+0.0i], [0.0+0.0i, 0.0+0.0i, 0.0+0.0i], [0.0+0.0i, 0.0+0.0i, 0.0+0.0i]] ("y")
      n24 = shared-variable "MGCC\\MGCC_StaEst.lvlib\\c_MGCC_StaEst_VOL"(w3950) -> ()  [unwired: 1 in, 1 out]
      n25 = mathscript code="if p_node == zero_t\noutput=true;\nelse\noutput=false;\nend"("zero_t"=w3944, "p_node"=w3949) -> ("output"=w3952:bool)  [unwired: 1 in, 1 out]
      n26 = Complex To Re/Im(x + iy=w3944) -> (x=w3951:dbl[][])  [unwired: 1 out]
      n27 = case shown="False" w3952 {
        tunnel: [w3953 w3955] -> w3945
        tunnel: [w3954 w3955] -> w3947
        tunnel: w3951 -> [_ w3955]
        tunnel: w3948 -> [w3954 _]
        tunnel: w3946 -> [w3953 _]
        frame False {
        }
        frame True {
        }
      }
      "VN" <- w3947
      "AN" <- w3945
      n28 = shared-variable "MGCC\\MGCC_StaEst.lvlib\\f_MGCC_StaEst_An"(w3945) -> ()  [unwired: 1 in, 1 out]
      n29 = shared-variable "MGCC\\MGCC_StaEst.lvlib\\f_MGCC_StaEst_Vn"(w3947) -> ()  [unwired: 1 in, 1 out]
    }
  }
